vi "Test Invert Transformation Matrix.vi"(11 "Test Case In":refnum<class "03_AR.lvclass">) -> (0 "error out":errorcluster, 3 "Test Case Out":refnum<class "03_AR.lvclass">)   [LabVIEW 2020, in "test.lvlib" / "03_AR.lvclass"]
uses:
  03_AR.lvclass
  usr/local/natinst/LabVIEW-2024-64/vi.lib/Astemes/LUnit/Test Case.lvclass
  ar/Roll-Pitch-Yaw.ctl
  <vilib>/Analysis/Matrix/Datatypes/RealMatrix.ctl
  <vilib>/Astemes/LUnit/Test Case.lvclass/Test Case.ctl
  4993e8ee-a06a-463a-9684-69129f64d5ce.vi
  <vilib>/Analysis/baseanly.llb/A x B.vi
  <vilib>/Analysis/baseanly.llb/A x Vector.vi
  ar/Transformation Matrix to Transform Components.vi
  ar/Transform Components to Transformation Matrix.vi
  <vilib>/Astemes/LUnit/Append Pass Result.vi
  <vilib>/Astemes/LUnit/Append Fail Result.vi
  <vilib>/Astemes/LUnit/Describe Comparison.vi
  4993e8ee-a06a-463a-9684-69129f64d5ce.vi/9c5d11cd-9439-4240-a1ee-d9baace9c924.vi
  <vilib>/Astemes/LUnit/Run In UI.vi
  <vilib>/Utility/error.llb/Clear Errors.vi
  <vilib>/Utility/error.llb/Error Cluster From Error Code.vi
  <vilib>/Analysis/Matrix/Numeric/Conversions/Array To Matrix.vi
  <vilib>/Analysis/Matrix/Numeric/Conversions/Array To Matrix - RA2.vi
  <vilib>/Analysis/baseanly.llb/Real Inverse Matrix.vi
  <vilib>/Astemes/LUnit/Describe Variant.vi
  <vilib>/Analysis/Matrix/Numeric/Subtract/Subtract.vi
  <vilib>/Analysis/Matrix/Numeric/Subtract/Subtract - RM,RM.vi
  <vilib>/Analysis/Matrix/Numeric/Absolute Value/Absolute Value.vi
  <vilib>/Analysis/Matrix/Numeric/Absolute Value/Absolute Value - RM.vi
  ar/ar.lvlib
  <vilib>/Analysis/NI_AALBase.lvlib
  <vilib>/Analysis/Matrix/NI_Matrix.lvlib
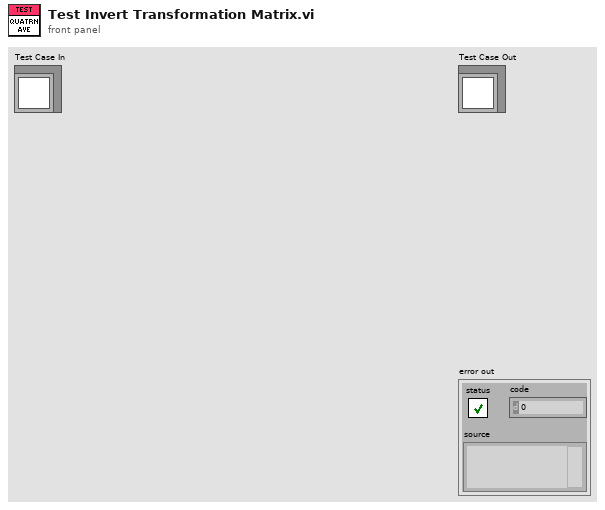
[diagram p1: front panel]
types:
  T1 = typedef "NI_Matrix.lvlib/RealMatrix.ctl" = dbl[][]
  T2 = typedef "ar.lvlib/Roll-Pitch-Yaw.ctl" = cluster{"roll":dbl, "pitch":dbl, "yaw":dbl}
  T3 = typedef "ar.lvlib/Quaternion.ctl" = cluster{"w":dbl, "x":dbl, "y":dbl, "z":dbl}
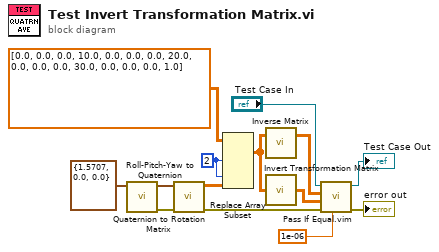
[diagram p0: block diagram]
diagram:
  w2 = 2 ("row N")
  n1 = call "Roll-Pitch-Yaw to Quaternion.vi"("Roll-Pitch-Yaw (rad)"=T2 {"roll"=1.5707, "pitch"=0.0, "yaw"=0.0}) -> ("error out"=w9:errorcluster, "Quaternion"=w10:T3)  [unwired: 9 in]
  n2 = call "Quaternion to Rotation Matrix.vi"("error in (no error)"=w9, "Quaternion"=w10) -> ("error out"=w6:errorcluster, "Rotation Matrix"=w4:T1)  [unwired: 8 in]
  n3 = Replace Array Subset(array=T1 [[0.0, 0.0, 0.0, 10.0], [0.0, 0.0, 0.0, 20.0], [0.0, 0.0, 0.0, 30.0], [0.0, 0.0, 0.0, 1.0]] ("Real Matrix"), new element=w4, index (dim 1)=w2, index (dim 3)=w2) -> (w3:T1)  [unwired: 2 in]
  n4 = call-poly <vilib>:"Inverse Matrix.vi"("Input Matrix"=w3) -> ("Inverse Matrix"=w8:T1)  [unwired: 1 in, 1 out]
  n5 = call "Invert Transformation Matrix.vi"("4x4 Transformation Matrix"=w3) -> ("Inverted 4x4 Transformation Matrix"=w7:T1)
  n6 = call "Pass If Equal.vim"("Delta"=1e-06, "error in (no error)"=w6, "Actual"=w7, "Expected"=w8, "LUnit Test Case In"="Test Case In") -> ("error out"=→"error out":errorcluster, "LUnit Test Case Out"=→"Test Case Out":refnum<class "03_AR.lvclass">)  [unwired: 5 in]
